vi "Read ActionVIType.vi"(8 "error in (no error)":errorcluster, 11 "ActionVI in":refnum<class "ActionVI.lvclass">) -> (0 "error out":errorcluster, 2 "Enum":T1, 3 "ActionVI out":refnum<class "ActionVI.lvclass">)   [LabVIEW 2015, in "ActionVI.lvclass"]
uses:
  ActionVI.lvclass
  Controls/ActionVITypes.ctl
  ActionVI.lvclass/ActionVI.ctl
  Configuration Tool.lvlib
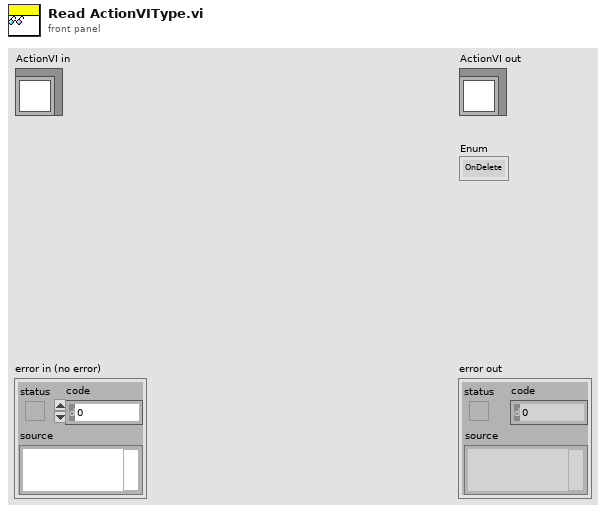
[diagram p1: front panel]
types:
  T1 = typedef "Configuration Tool.lvlib/ActionVITypes.ctl" = enum16{"OnDelete", "OnLoad", "OnPaste", "OnTargetTypeChange", "OnDeleteRequest", "OnCompile", "OnSystemShutdown", "OnSave", "OnDownload"}
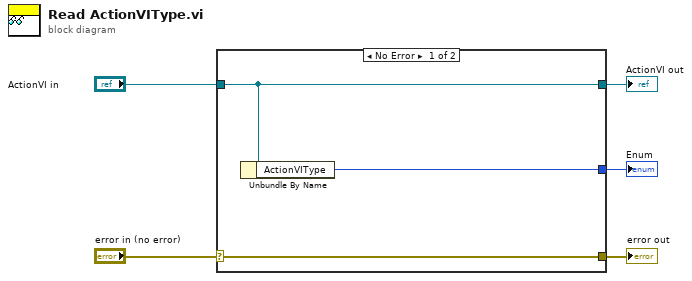
[diagram p0: block diagram]
diagram:
  n1 = case shown="No Error" "error in (no error)" {
    selector: "error in (no error)" -> [w8 w9]
    tunnel: [w8 w9] -> w4
    tunnel: [w7 w10] -> w2
    tunnel: "ActionVI in" -> [w7 w10]
    tunnel: [w6 _] -> w1
    frame No Error {
      n2 = Unbundle By Name(w7) -> ("ActionVIType"=w6:T1)
    }
    frame Error {
    }
  }
  "error out" <- w4
  "ActionVI out" <- w2
  "Enum" <- w1
